vi "FindDependency(byKey).vi"(8 "error in (no error)":errorcluster, 9 "Search Key (Name)":T1, 10 "Key":string, 11 "SMO in":refnum<class "SMO.lvclass">) -> (0 "error out":errorcluster, 1 "Found?":bool, 2 "Dependency":refnum<class "SMO.lvclass">, 3 "SMO dup":refnum<class "SMO.lvclass">)   [LabVIEW 2013, in "SMO.lvclass"]
uses:
  SMO.lvclass
  Typedefs/Search Key.ctl
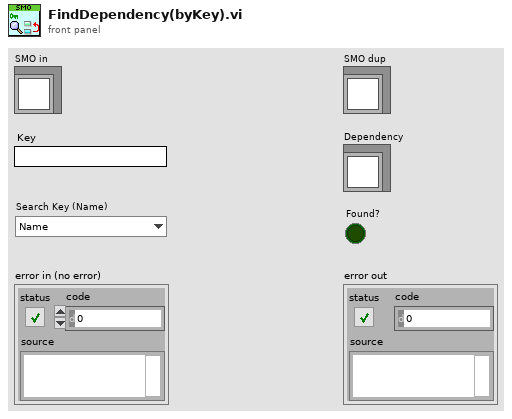
[diagram p1: front panel]
types:
  T1 = typedef "SMO.lvclass/Search Key.ctl" = enum16{"Name", "GUID", "Qualified Name", "Subsystem Path", "Configuration Path"}
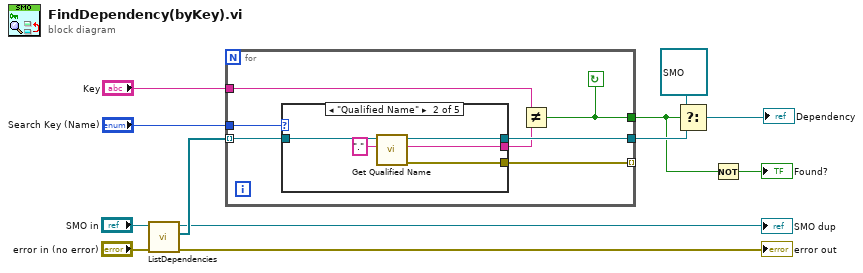
[diagram p0: block diagram]
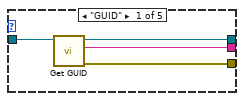
[diagram p2: hidden frame]
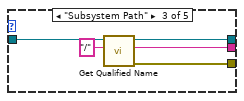
[diagram p3: hidden frame]
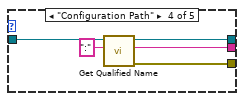
[diagram p4: hidden frame]
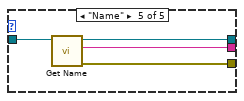
[diagram p5: hidden frame]
diagram:
  n1 = call "ListDependencies.vi"("error in (no error)"="error in (no error)", "SMO in"="SMO in") -> ("error out"=→"error out":errorcluster, "[Dependencies]"=w11:refnum<class "SMO.lvclass">[], "SMO out"=→"SMO dup":refnum<class "SMO.lvclass">)  [unwired: 6 in, 1 out]
  n2 = for {
    tunnel: w11 -> [w19] mode=indexing
    tunnel: [w18] -> w6
    tunnel: "Key" -> [w14]
    tunnel: [w16] -> w4
    tunnel: [w15] -> _ mode=indexing
    tunnel: "Search Key (Name)" -> [w13]
    stop <- w16 continue-if-true
    n3 = case shown="\"Qualified Name\"" w13 {
      tunnel: w19 -> [w23 w28 w33 w38 w42]
      tunnel: [w22 w27 w32 w37 w41] -> w18
      tunnel: [w21 w26 w31 w36 w40] -> w17
      tunnel: [w20 w25 w30 w35 w39] -> w15
      frame "GUID" {
        n4 = call "Get GUID.vi"("SMO"=w23) -> ("error out"=w20:errorcluster, "GUID"=w21:string, "SMO out"=w22:refnum<class "SMO.lvclass">)  [unwired: 8 in]
      }
      frame "Qualified Name" {
        n5 = call "Get Qualified Name.vi"("separator (dot)"=".", "SMO"=w28) -> ("error out"=w25:errorcluster, "Qualified Name"=w26:string, "SMO out"=w27:refnum<class "SMO.lvclass">)  [unwired: 7 in]
      }
      frame "Subsystem Path" {
        n6 = call "Get Qualified Name.vi"("separator (dot)"="/", "SMO"=w33) -> ("error out"=w30:errorcluster, "Qualified Name"=w31:string, "SMO out"=w32:refnum<class "SMO.lvclass">)  [unwired: 7 in]
      }
      frame "Configuration Path" {
        n7 = call "Get Qualified Name.vi"("separator (dot)"=":", "SMO"=w38) -> ("error out"=w35:errorcluster, "Qualified Name"=w36:string, "SMO out"=w37:refnum<class "SMO.lvclass">)  [unwired: 7 in]
      }
      frame "Name" {
        n8 = call "Get Name.vi"("SMO"=w42) -> ("error out"=w39:errorcluster, "Name"=w40:string, "SMO out"=w41:refnum<class "SMO.lvclass">)  [unwired: 8 in]
      }
    }
    n9 = Not Equal?(x=w14, y=w17) -> (x != y?=w16:bool)
  }
  n10 = Select(t=refnum<class "SMO.lvclass"> refnum ("f"), s=w4, f=w6) -> (s? t:f=→"Dependency":refnum<class "SMO.lvclass">)
  n11 = Not(x=w4) -> (.not. x?=→"Found?":bool)
